vi "Init.vi"(4 "Rename":string, 6 "Name":string, 9 "Project:Active Project":refnum<vi>) -> (3 "Script out":refnum<class "Script.lvclass">)   [LabVIEW 2021, in "_Rename.lvlib" / "Script.lvlib" / "Script.lvclass"]
uses:
  Script.lvclass
  Script.lvclass/Script.ctl
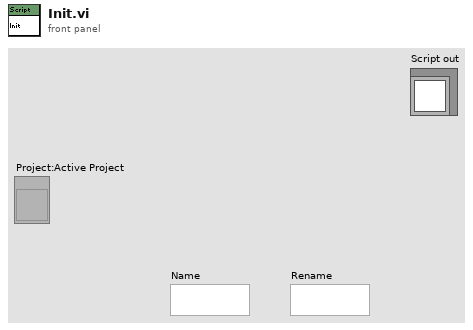
[diagram p1: front panel]
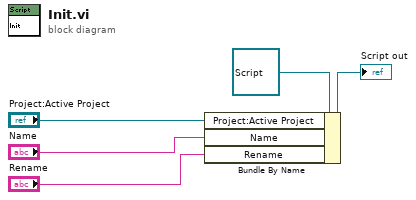
[diagram p0: block diagram]
diagram:
  n1 = Bundle By Name(cluster=refnum<class "Script.lvclass"> refnum ("Script out"), "Project:Active Project"="Project:Active Project", "Name"="Name", "Rename"="Rename") -> (→"Script out":refnum<class "Script.lvclass">)
